vi "Get Channel Attribute String Wrapper.vi"(0 "Task map in":map{string, refnum<k21>}(c390), 5 "Message Data in":T2, 11 "error in (no error)":errorcluster) -> (4 "Task map out":map{string, refnum<k21>}(c390), 6 "Message Data out":T1, 15 "error out":errorcluster)   [LabVIEW 2021, in "NI DAQmx_wrapper.lvlib"]
uses:
  NI DAQmx_wrapper.lvlib
  NI DAQmx_server/RPC Messages/nidaqmx_grpc_GetChanAttributeStringRequest.ctl
  NI DAQmx_server/RPC Messages/nidevice_grpc_Session_session/nidevice_grpc_Session_session.lvclass
  NI DAQmx_server/RPC Messages/nidaqmx_grpc_GetChanAttributeStringRequest_attribute_enum/nidaqmx_grpc_GetChanAttributeStringRequest_attribute_enum.lvclass
  NI DAQmx_server/RPC Messages/nidevice_grpc_Session.ctl
  NI DAQmx_server/RPC Messages/nidaqmx_grpc_GetChanAttributeStringResponse.ctl
  NI DAQmx_server/RPC Messages/nidaqmx_grpc_GetChanAttributeStringRequest_attribute_enum/nidaqmx_grpc_GetChanAttributeStringRequest_attribute_enum.lvclass/nidaqmx_grpc_GetChanAttributeStringRequest_attribute_enum.ctl
  NI DAQmx_server/RPC Messages/nidevice_grpc_Session_session/nidevice_grpc_Session_session.lvclass/nidevice_grpc_Session_session.ctl
  <resource>/objmgr/daqmx.rc
  NI DAQmx_server/NI DAQmx_server.lvlib
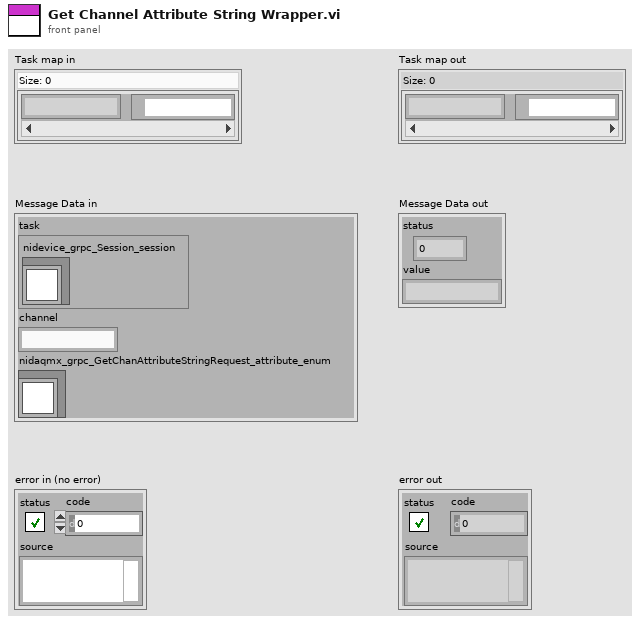
[diagram p1: front panel]
types:
  T1 = typedef "NI DAQmx_server.lvlib/nidaqmx_grpc_GetChanAttributeStringResponse.ctl" = cluster{"status":i32, "value":string}
  T2 = typedef "NI DAQmx_server.lvlib/nidaqmx_grpc_GetChanAttributeStringRequest.ctl" = cluster{"task":T3, "channel":string, "nidaqmx_grpc_GetChanAttributeStringRequest_attribute_enum":refnum<class "nidaqmx_grpc_GetChanAttributeStringRequest_attribute_enum.lvclass">}
  T3 = typedef "NI DAQmx_server.lvlib/nidevice_grpc_Session.ctl" = cluster{"nidevice_grpc_Session_session":refnum<class "nidevice_grpc_Session_session.lvclass">}
  T4 = typedef "NI DAQmx_server.lvlib/nidaqmx_grpc_ChannelStringAttribute.ctl" = enum32{"CHANNEL_STRING_ATTRIBUTE_UNSPECIFIED", "CHANNEL_ATTRIBUTE_CI_CTR_TIMEBASE_SRC", "CHANNEL_ATTRIBUTE_CO_CTR_TIMEBASE_SRC", "CHANNEL_ATTRIBUTE_AI_THRMCPL_CJC_CHAN", "CHANNEL_ATTRIBUTE_CI_GPS_SYNC_SRC", "CHANNEL_ATTRIBUTE_AO_CUSTOM_SCALE_NAME", "CHANNEL_ATTRIBUTE_AI_CUSTOM_SCALE_NAME", "CHANNEL_ATTRIBUTE_CI_CUSTOM_SCALE_NAME", "CHANNEL_ATTRIBUTE_CI_FREQ_TERM", "CHANNEL_ATTRIBUTE_CI_PERIOD_TERM", "CHANNEL_ATTRIBUTE_CI_PULSE_WIDTH_TERM", "CHANNEL_ATTRIBUTE_CI_TWO_EDGE_SEP_FIRST_TERM", "CHANNEL_ATTRIBUTE_CI_TWO_EDGE_SEP_SECOND_TERM", "CHANNEL_ATTRIBUTE_CI_SEMI_PERIOD_TERM", "CHANNEL_ATTRIBUTE_CI_COUNT_EDGES_TERM", "CHANNEL_ATTRIBUTE_CO_PULSE_TERM", "CHANNEL_ATTRIBUTE_PHYSICAL_CHAN_NAME", "CHANNEL_ATTRIBUTE_CHAN_DESCR", "CHANNEL_ATTRIBUTE_AI_INPUT_SRC", "CHANNEL_ATTRIBUTE_CI_ENCODER_A_INPUT_TERM", "CHANNEL_ATTRIBUTE_CI_ENCODER_B_INPUT_TERM", "CHANNEL_ATTRIBUTE_CI_ENCODER_Z_INPUT_TERM", "CHANNEL_ATTRIBUTE_AI_TEDS_UNITS", "CHANNEL_ATTRIBUTE_CI_COUNT_EDGES_DIR_TERM", "CHANNEL_ATTRIBUTE_CI_FREQ_DIG_FLTR_TIMEBASE_SRC", "CHANNEL_ATTRIBUTE_CI_PERIOD_DIG_FLTR_TIMEBASE_SRC", "CHANNEL_ATTRIBUTE_CI_COUNT_EDGES_COUNT_DIR_DIG_FLTR_TIMEBASE_SRC", "CHANNEL_ATTRIBUTE_CI_COUNT_EDGES_DIG_FLTR_TIMEBASE_SRC", "CHANNEL_ATTRIBUTE_CI_ENCODER_A_INPUT_DIG_FLTR_TIMEBASE_SRC", "CHANNEL_ATTRIBUTE_CI_ENCODER_B_INPUT_DIG_FLTR_TIMEBASE_SRC", "CHANNEL_ATTRIBUTE_CI_ENCODER_Z_INPUT_DIG_FLTR_TIMEBASE_SRC", "CHANNEL_ATTRIBUTE_CI_PULSE_WIDTH_DIG_FLTR_TIMEBASE_SRC", "CHANNEL_ATTRIBUTE_CI_TWO_EDGE_SEP_FIRST_DIG_FLTR_TIMEBASE_SRC", "CHANNEL_ATTRIBUTE_CI_TWO_EDGE_SEP_SECOND_DIG_FLTR_TIMEBASE_SRC", "CHANNEL_ATTRIBUTE_CI_SEMI_PERIOD_DIG_FLTR_TIMEBASE_SRC", "CHANNEL_ATTRIBUTE_AO_DAC_REF_EXT_SRC", "CHANNEL_ATTRIBUTE_AO_DAC_OFFSET_EXT_SRC", "CHANNEL_ATTRIBUTE_CI_CTR_TIMEBASE_DIG_FLTR_TIMEBASE_SRC", "CHANNEL_ATTRIBUTE_CO_CTR_TIMEBASE_DIG_FLTR_TIMEBASE_SRC", "CHANNEL_ATTRIBUTE_AI_CHAN_CAL_OPERATOR_NAME", "CHANNEL_ATTRIBUTE_AI_CHAN_CAL_DESC", "CHANNEL_ATTRIBUTE_DI_DIG_FLTR_TIMEBASE_SRC", "CHANNEL_ATTRIBUTE_CI_PULSE_FREQ_TERM", "CHANNEL_ATTRIBUTE_CI_PULSE_FREQ_DIG_FLTR_TIMEBASE_SRC", "CHANNEL_ATTRIBUTE_CI_PULSE_TIME_TERM", "CHANNEL_ATTRIBUTE_CI_PULSE_TIME_DIG_FLTR_TIMEBASE_SRC", "CHANNEL_ATTRIBUTE_CI_PULSE_TICKS_TERM", "CHANNEL_ATTRIBUTE_CI_PULSE_TICKS_DIG_FLTR_TIMEBASE_SRC", "CHANNEL_ATTRIBUTE_CI_COUNT_EDGES_COUNT_RESET_TERM", "CHANNEL_ATTRIBUTE_CI_COUNT_EDGES_COUNT_RESET_DIG_FLTR_TIMEBASE_SRC", "CHANNEL_ATTRIBUTE_AI_ROSETTE_STRAIN_GAGE_STRAIN_CHANS", "CHANNEL_ATTRIBUTE_CI_TIMESTAMP_TERM", "CHANNEL_ATTRIBUTE_NAV_CUSTOM_SCALE_NAME", "CHANNEL_ATTRIBUTE_CI_DUTY_CYCLE_TERM", "CHANNEL_ATTRIBUTE_CI_DUTY_CYCLE_DIG_FLTR_TIMEBASE_SRC", "CHANNEL_ATTRIBUTE_CI_VELOCITY_ENCODER_A_INPUT_TERM", "CHANNEL_ATTRIBUTE_CI_VELOCITY_ENCODER_A_INPUT_DIG_FLTR_TIMEBASE_SRC", "CHANNEL_ATTRIBUTE_CI_VELOCITY_ENCODER_B_INPUT_TERM", "CHANNEL_ATTRIBUTE_CI_VELOCITY_ENCODER_B_INPUT_DIG_FLTR_TIMEBASE_SRC", "CHANNEL_ATTRIBUTE_CI_COUNT_EDGES_GATE_TERM", "CHANNEL_ATTRIBUTE_CI_COUNT_EDGES_GATE_DIG_FLTR_TIMEBASE_SRC"}
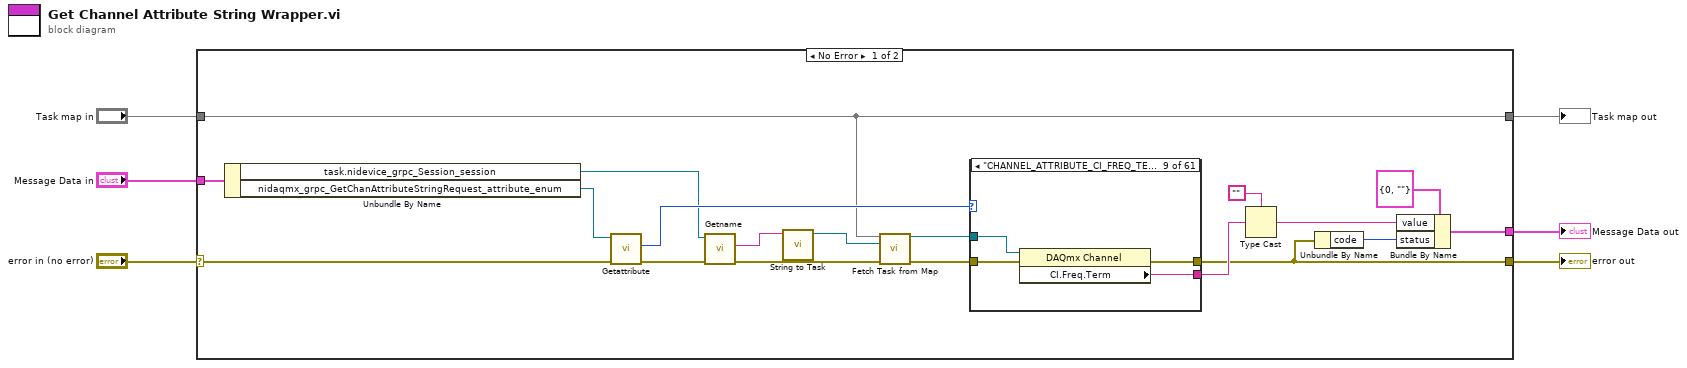
[diagram p0: block diagram]
diagram:
  n1 = case shown="No Error" "error in (no error)" {
    selector: "error in (no error)" -> [w24 w91]
    tunnel: [w10 w91] -> w5
    tunnel: "Task map in" -> [w14 w90]
    tunnel: [w14 w90] -> w3
    tunnel: "Message Data in" -> [w25 _]
    tunnel: [w7 _] -> w1
    frame No Error {
      n2 = Unbundle By Name(w25) -> ("task.nidevice_grpc_Session_session"=w16:refnum<class "nidevice_grpc_Session_session.lvclass">, "nidaqmx_grpc_GetChanAttributeStringRequest_attribute_enum"=w23:refnum<class "nidaqmx_grpc_GetChanAttributeStringRequest_attribute_enum.lvclass">)
      n3 = call "Getattribute.vi"("error in (no error)"=w24, "OneOfTemplate in"=w23) -> ("error out"=w18:errorcluster, "Get_Val"=w22:T4)  [unwired: 7 in, 1 out]
      n4 = call "Getname.vi"("error in (no error)"=w18, "OneOfTemplate in"=w16) -> ("error out"=w21:errorcluster, "Get_Val"=w20:string)  [unwired: 7 in, 1 out]
      n5 = call "String to Task.vi"("Get_Val"=w20) -> ("Refnum out"=w19:refnum<k21>)  [unwired: 10 in]
      n6 = call "Fetch Task from Map.vi"("Task map in"=w14, "Task in"=w19, "error in (no error)"=w21) -> ("Task out"=w15:refnum<k21>, "error out"=w17:errorcluster)  [unwired: 11 in]
      n7 = case shown="\"CHANNEL_ATTRIBUTE_CI_FREQ_TERM\"" w22 {
        tunnel: w17 -> [w26 w27 w28 w29 w30 w31 w32 w33 w37 w38 w39 w40 w41 w42 w43 w44 w45 w46 w47 w48 w49 w50 w51 w52 w53 w54 w55 w56 w57 w58 w59 w60 w61 w62 w63 w64 w65 w66 w67 w68 w69 w70 w71 w72 w73 w74 w75 w76 w77 w78 w79 w80 w81 w82 w83 w84 w85 w86 w87 w88 w89]
        tunnel: [w26 w27 w28 w29 w30 w31 w32 w33 w36 w38 w39 w40 w41 w42 w43 w44 w45 w46 w47 w48 w49 w50 w51 w52 w53 w54 w55 w56 w57 w58 w59 w60 w61 w62 w63 w64 w65 w66 w67 w68 w69 w70 w71 w72 w73 w74 w75 w76 w77 w78 w79 w80 w81 w82 w83 w84 w85 w86 w87 w88 w89] -> w10
        tunnel: w15 -> [_ _ _ _ _ _ _ _ w35 _ _ _ _ _ _ _ _ _ _ _ _ _ _ _ _ _ _ _ _ _ _ _ _ _ _ _ _ _ _ _ _ _ _ _ _ _ _ _ _ _ _ _ _ _ _ _ _ _ _ _ _]
        tunnel: [_ _ _ _ _ _ _ _ w34 _ _ _ _ _ _ _ _ _ _ _ _ _ _ _ _ _ _ _ _ _ _ _ _ _ _ _ _ _ _ _ _ _ _ _ _ _ _ _ _ _ _ _ _ _ _ _ _ _ _ _ _] -> w13
        frame "CHANNEL_STRING_ATTRIBUTE_UNSPECIFIED", Default {
        }
        frame "CHANNEL_ATTRIBUTE_CI_CTR_TIMEBASE_SRC" {
        }
        frame "CHANNEL_ATTRIBUTE_CO_CTR_TIMEBASE_SRC" {
        }
        frame "CHANNEL_ATTRIBUTE_AI_THRMCPL_CJC_CHAN" {
        }
        frame "CHANNEL_ATTRIBUTE_CI_GPS_SYNC_SRC" {
        }
        frame "CHANNEL_ATTRIBUTE_AO_CUSTOM_SCALE_NAME" {
        }
        frame "CHANNEL_ATTRIBUTE_AI_CUSTOM_SCALE_NAME" {
        }
        frame "CHANNEL_ATTRIBUTE_CI_CUSTOM_SCALE_NAME" {
        }
        frame "CHANNEL_ATTRIBUTE_CI_FREQ_TERM" {
          n8 = property class="DAQmx Channel"(reference=w35, error in=w37) -> (error out=w36:errorcluster, "CI.Freq.Term"=w34:tag)  [unwired: 1 out]
        }
        frame "CHANNEL_ATTRIBUTE_CI_PERIOD_TERM" {
        }
        frame "CHANNEL_ATTRIBUTE_CI_PULSE_WIDTH_TERM" {
        }
        frame "CHANNEL_ATTRIBUTE_CI_TWO_EDGE_SEP_FIRST_TERM" {
        }
        frame "CHANNEL_ATTRIBUTE_CI_TWO_EDGE_SEP_SECOND_TERM" {
        }
        frame "CHANNEL_ATTRIBUTE_CI_SEMI_PERIOD_TERM" {
        }
        frame "CHANNEL_ATTRIBUTE_CI_COUNT_EDGES_TERM" {
        }
        frame "CHANNEL_ATTRIBUTE_CO_PULSE_TERM" {
        }
        frame "CHANNEL_ATTRIBUTE_PHYSICAL_CHAN_NAME" {
        }
        frame "CHANNEL_ATTRIBUTE_CHAN_DESCR" {
        }
        frame "CHANNEL_ATTRIBUTE_AI_INPUT_SRC" {
        }
        frame "CHANNEL_ATTRIBUTE_CI_ENCODER_A_INPUT_TERM" {
        }
        frame "CHANNEL_ATTRIBUTE_CI_ENCODER_B_INPUT_TERM" {
        }
        frame "CHANNEL_ATTRIBUTE_CI_ENCODER_Z_INPUT_TERM" {
        }
        frame "CHANNEL_ATTRIBUTE_AI_TEDS_UNITS" {
        }
        frame "CHANNEL_ATTRIBUTE_CI_COUNT_EDGES_DIR_TERM" {
        }
        frame "CHANNEL_ATTRIBUTE_CI_FREQ_DIG_FLTR_TIMEBASE_SRC" {
        }
        frame "CHANNEL_ATTRIBUTE_CI_PERIOD_DIG_FLTR_TIMEBASE_SRC" {
        }
        frame "CHANNEL_ATTRIBUTE_CI_COUNT_EDGES_COUNT_DIR_DIG_FLTR_TIMEBASE_SRC" {
        }
        frame "CHANNEL_ATTRIBUTE_CI_COUNT_EDGES_DIG_FLTR_TIMEBASE_SRC" {
        }
        frame "CHANNEL_ATTRIBUTE_CI_ENCODER_A_INPUT_DIG_FLTR_TIMEBASE_SRC" {
        }
        frame "CHANNEL_ATTRIBUTE_CI_ENCODER_B_INPUT_DIG_FLTR_TIMEBASE_SRC" {
        }
        frame "CHANNEL_ATTRIBUTE_CI_ENCODER_Z_INPUT_DIG_FLTR_TIMEBASE_SRC" {
        }
        frame "CHANNEL_ATTRIBUTE_CI_PULSE_WIDTH_DIG_FLTR_TIMEBASE_SRC" {
        }
        frame "CHANNEL_ATTRIBUTE_CI_TWO_EDGE_SEP_FIRST_DIG_FLTR_TIMEBASE_SRC" {
        }
        frame "CHANNEL_ATTRIBUTE_CI_TWO_EDGE_SEP_SECOND_DIG_FLTR_TIMEBASE_SRC" {
        }
        frame "CHANNEL_ATTRIBUTE_CI_SEMI_PERIOD_DIG_FLTR_TIMEBASE_SRC" {
        }
        frame "CHANNEL_ATTRIBUTE_AO_DAC_REF_EXT_SRC" {
        }
        frame "CHANNEL_ATTRIBUTE_AO_DAC_OFFSET_EXT_SRC" {
        }
        frame "CHANNEL_ATTRIBUTE_CI_CTR_TIMEBASE_DIG_FLTR_TIMEBASE_SRC" {
        }
        frame "CHANNEL_ATTRIBUTE_CO_CTR_TIMEBASE_DIG_FLTR_TIMEBASE_SRC" {
        }
        frame "CHANNEL_ATTRIBUTE_AI_CHAN_CAL_OPERATOR_NAME" {
        }
        frame "CHANNEL_ATTRIBUTE_AI_CHAN_CAL_DESC" {
        }
        frame "CHANNEL_ATTRIBUTE_DI_DIG_FLTR_TIMEBASE_SRC" {
        }
        frame "CHANNEL_ATTRIBUTE_CI_PULSE_FREQ_TERM" {
        }
        frame "CHANNEL_ATTRIBUTE_CI_PULSE_FREQ_DIG_FLTR_TIMEBASE_SRC" {
        }
        frame "CHANNEL_ATTRIBUTE_CI_PULSE_TIME_TERM" {
        }
        frame "CHANNEL_ATTRIBUTE_CI_PULSE_TIME_DIG_FLTR_TIMEBASE_SRC" {
        }
        frame "CHANNEL_ATTRIBUTE_CI_PULSE_TICKS_TERM" {
        }
        frame "CHANNEL_ATTRIBUTE_CI_PULSE_TICKS_DIG_FLTR_TIMEBASE_SRC" {
        }
        frame "CHANNEL_ATTRIBUTE_CI_COUNT_EDGES_COUNT_RESET_TERM" {
        }
        frame "CHANNEL_ATTRIBUTE_CI_COUNT_EDGES_COUNT_RESET_DIG_FLTR_TIMEBASE_SRC" {
        }
        frame "CHANNEL_ATTRIBUTE_AI_ROSETTE_STRAIN_GAGE_STRAIN_CHANS" {
        }
        frame "CHANNEL_ATTRIBUTE_CI_TIMESTAMP_TERM" {
        }
        frame "CHANNEL_ATTRIBUTE_NAV_CUSTOM_SCALE_NAME" {
        }
        frame "CHANNEL_ATTRIBUTE_CI_DUTY_CYCLE_TERM" {
        }
        frame "CHANNEL_ATTRIBUTE_CI_DUTY_CYCLE_DIG_FLTR_TIMEBASE_SRC" {
        }
        frame "CHANNEL_ATTRIBUTE_CI_VELOCITY_ENCODER_A_INPUT_TERM" {
        }
        frame "CHANNEL_ATTRIBUTE_CI_VELOCITY_ENCODER_A_INPUT_DIG_FLTR_TIMEBASE_SRC" {
        }
        frame "CHANNEL_ATTRIBUTE_CI_VELOCITY_ENCODER_B_INPUT_TERM" {
        }
        frame "CHANNEL_ATTRIBUTE_CI_VELOCITY_ENCODER_B_INPUT_DIG_FLTR_TIMEBASE_SRC" {
        }
        frame "CHANNEL_ATTRIBUTE_CI_COUNT_EDGES_GATE_TERM" {
        }
        frame "CHANNEL_ATTRIBUTE_CI_COUNT_EDGES_GATE_DIG_FLTR_TIMEBASE_SRC" {
        }
      }
      n9 = Type Cast(type="", x=w13) -> (*(type *) &x=w8:string)
      n10 = Unbundle By Name(w10) -> ("code"=w11:i32)
      n11 = Bundle By Name(cluster=T1 {"status"=0, "value"=""} ("Message Data"), "value"=w8, "status"=w11) -> (w7:T1)
    }
    frame Error {
    }
  }
  "error out" <- w5
  "Task map out" <- w3
  "Message Data out" <- w1
